vi "Find Port by Id.vi"(8 "error in":errorcluster, 10 "portId":i32, 11 "ports ref in":T1 format="%.0x") -> (0 "error out":errorcluster, 2 "ports ref out":T1 format="%.0x", 3 "ports ref out":T1=18446744073709551615 format="%.0x", 4 "found?":bool)   [LabVIEW 2020, in "AIM ARINC 664 Scripting.lvlib"]
uses:
  AIM ARINC 664 Scripting.lvlib
  Constants.vi
  <vilib>/NI VeriStand/Custom Device Tools/Custom Device Utility Library/Custom Device Utility Library.lvlib
  <vilib>/NI VeriStand/Custom Device API/Custom Device API.lvlib
  <vilib>/NI VeriStand/Custom Device Tools/Custom Device Utility Library/NI VeriStand - Search for All Items by GUID.vi
  <vilib>/NI VeriStand/Custom Device API/Get Item Property (U32).vi
  <vilib>/NI VeriStand/Custom Device API/Custom Device Item Ref.ctl
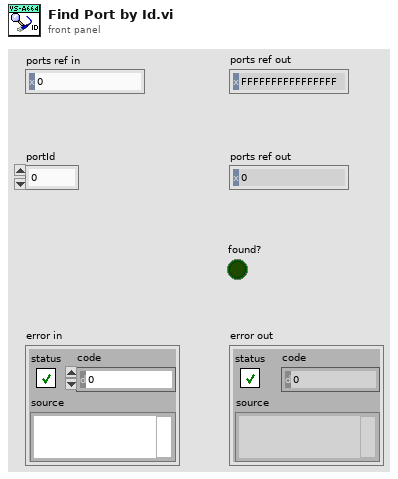
[diagram p1: front panel]
types:
  T1 = typedef "Custom Device API.lvlib/Custom Device Item Ref.ctl" = u64
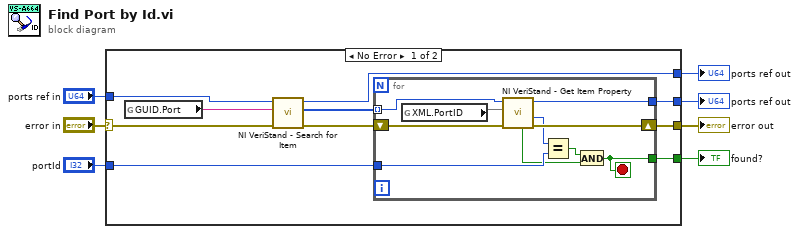
[diagram p0: block diagram]
diagram:
  n1 = case shown="No Error" "error in" {
    selector: "error in" -> [w15 w29]
    tunnel: "ports ref in" -> [w16 w28]
    tunnel: [w10 w29] -> w6
    tunnel: "portId" -> [w9 _]
    tunnel: [w13 w28] -> w3
    tunnel: [w11 _] -> w2
    tunnel: [w8 _] -> w1
    frame No Error {
      n2 = global read "Constants.vi" "GUID.Port"() -> (w17:string)
      n3 = call-poly <vilib>:"NI VeriStand - Search for Item.vi"("error in"=w15, "Item GUID"=w17, "Section Ref in"=w16) -> ("error out"=w14:errorcluster, "Item Refs"=w12:T1[], "Section Ref out"=w13:T1)  [unwired: 5 in, 1 out]
      n4 = for {
        shift-right: [w23] -> w10
        shift-left: w14 -> [w27]
        tunnel: w12 -> [w26] mode=indexing
        tunnel: [w24] -> w11
        tunnel: w9 -> [w21]
        tunnel: [w18] -> w8
        stop <- w18 stop-if-true
        n5 = global read "Constants.vi" "XML.PortID"() -> (w25)
        n6 = call-poly <vilib>:"NI VeriStand - Get Item Property.vi"("error in (no error)"=w27, "Property Name"=w25, "Item Ref in"=w26) -> ("error out"=w23:errorcluster, "Value"=w22:u32, "Item Ref out"=w24:T1, "Found?"=w19:bool)  [unwired: 5 in]
        n7 = Equal?(x=w22, y=w21) -> (x = y?=w20:bool)
        n8 = And(x=w20, y=w19) -> (x .and. y?=w18:bool)
      }
    }
    frame Error {
    }
  }
  "error out" <- w6
  "ports ref out" <- w2
  "found?" <- w1
  "ports ref out" <- w3
